vi "IR2100_get_rdg.vi"(1 "Address":T1) -> (3 "Comment":string, 5 "Reading":dbl format="%.3f")   [LabVIEW 2017]
uses:
  ADAM Client/Sub VIs/ADAM Controls/Address.ctl
  <vilib>/Instr/serial.llb/serpConfig.vi
  <vilib>/Plasmionique/MB Master/MB Master.lvlib
  <vilib>/Plasmionique/MB Master/MB_Master_Serial/MB_Master_Serial.lvclass
  Applications/National Instruments/LabVIEW 2017 64-bit/vi.lib/Plasmionique/MB Master/MB_Master/MB_Master.lvclass
panel:
  out "Results (binary)":u16[](array[numeric])
  out "error out":errorcluster
  out "Channel":u16(ring) items=["Current Value", "Mode", "Status", "Gas type", "Unit type", "Version", "Gain", "Disable LED", "Solenoid I/O", "Address", "Ratio", "Baud Rate", "Data Format", "Not Used", "Not Used", "Not Used", "Not Used", "Not Used", "Not Used", "Not Used", "Not Used", "Not Used", "Not Used", "Not Used", "Not Used", "Not Used", "Not Used", "Not Used", "Not Used", "Not Used", "Not Used", "Not Used", "# Rcv Errors", "% Activity Rate", "# Function Err", "# Start Errors", "# Register Err.", "# CRC hi Errors", "# CRC lo Errors", "# Overrun Err.", "# Noise Errors", "# Framing Err", "Not Used", "Not Used", "Not Used", "Clear Errors"]
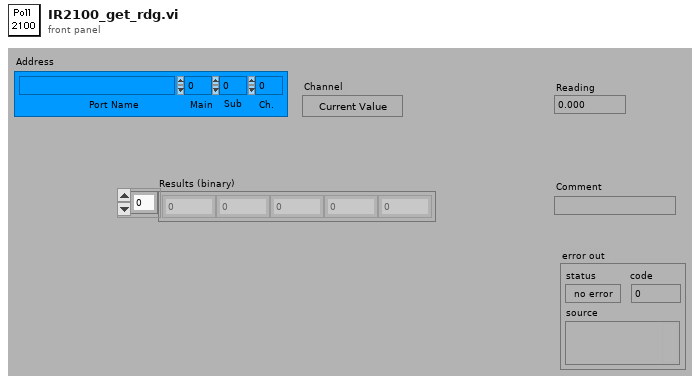
[diagram p1: front panel]
types:
  T1 = typedef "Address.ctl" = cluster{"Main":i32, "Ch.":i32, "Sub":i32, "Port Name":string}
  T2 = cluster{"baud rate (bps)":u32, "stop bits":u16, "parity":u16, "flow control":u16, "timeout":u32, "retries":i32}
  T3 = enum16{"01 Read digital output status", "02 Read digital input status", "03 Read output registers", "04 Read input registers", "05 Write single digital output", "06 Write single output register", "15 Write multiple digital outputs", "16 Write multiple output registers"}
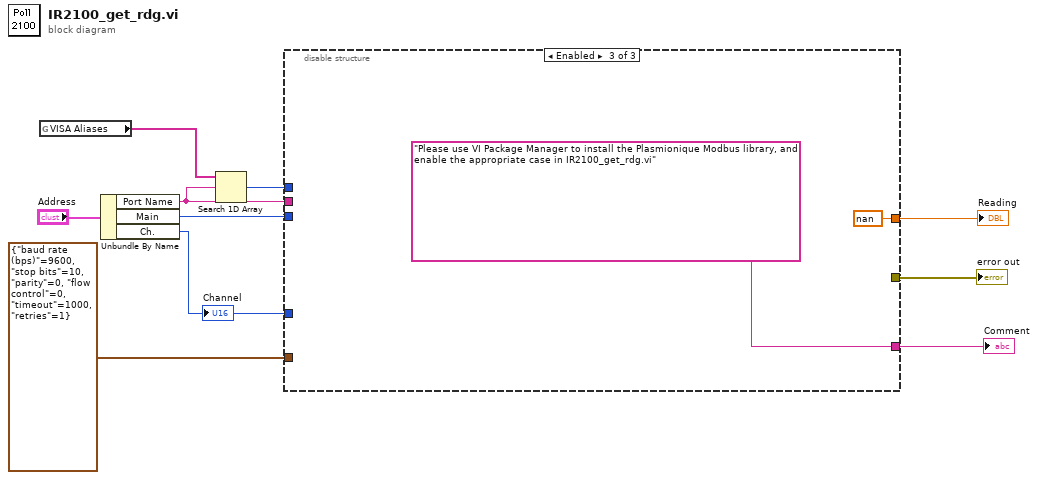
[diagram p0: block diagram]
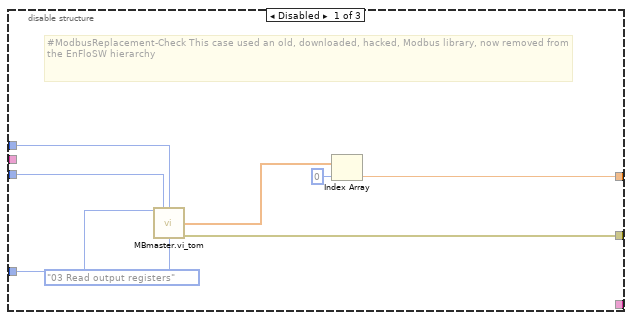
[diagram p2: hidden frame]
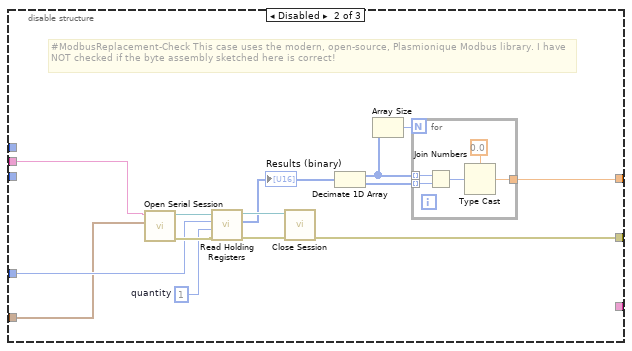
[diagram p3: hidden frame]
diagram:
  n1 = global read "serpConfig.vi" "VISA Aliases"() -> (w8:string[])
  n2 = Unbundle By Name("Address") -> ("Port Name"=w3:string, "Main"=w6:i32, "Ch."=w5:i32)
  "Channel" <- w5
  n3 = Search 1D Array(1D array=w8, element=w3) -> (index of element=w7:i32)  [unwired: 1 out]
  n4 = disable-structure shown="Enabled" {
    disable-tunnel: [w15 w20 nan ("Reading")] -> w10
    disable-tunnel: w7 -> [w14 _ _]
    disable-tunnel: w6 -> [w13 _ _]
    disable-tunnel: w5 -> [w12 w26 _]
    disable-tunnel: [w11 w30 _] -> w4
    disable-tunnel: w3 -> [_ w29 _]
    disable-tunnel: T2 {"baud rate (bps)"=9600, "stop bits"=10, "parity"=0, "flow control"=0, "timeout"=1000, "retries"=1} ("Serial Config") -> [_ w19 _]
    disable-tunnel: [_ _ "Please use VI Package Manager to install the Plasmionique Modbus library, and enable the appropriate case in IR2100_get_rdg.vi"] -> w1
    frame Disabled {
      # "#ModbusReplacement-Check This case used an old, downloaded, hacked, Modbus library, now removed from the EnFloSW hierarchy"
      n5 = call "MBmaster.vi_tom.vi"("Register address (0)"=w12, "Modbus address (1)"=w13, "port number"=w14, "ModBus Function"=T3."03 Read output registers") -> ("Process values"=w17:dbl[], "error out"=w11:errorcluster)  [unwired: 5 in, 5 out]
      n6 = Index Array(array=w17, index=0) -> (element=w15:dbl)
    }
    frame Disabled {
      w25 = u16 1  # quantity
      # "#ModbusReplacement-Check This case uses the modern, open-source, Plasmionique Modbus library. I have NOT checked if the byte assembly sketched here is correct!"
      n7 = call <vilib>:"Open Serial Session.vi"("Serial Config"=w19, "VISA Resource"=w29) -> ("Error out"=w32:errorcluster, "MB_Serial session"=w28:refnum<class "MB_Master_Serial.lvclass">)  [unwired: 8 in]
      n8 = call <vilib>:"Read Holding Registers.vi"("error in (no error)"=w32, "quantity"=w25, "starting address"=w26, "MB session in"=w28) -> ("error out"=w31:errorcluster, "Registers"=w21:u16[], "MB session out"=w27:refnum<class "MB_Master_Serial.lvclass">)  [unwired: 5 in]
      "Results (binary)" <- w21
      n9 = call-dynamic "Close Session.vi"("error in (no error)"=w31, "MB_Serial session"=w27) -> ("error out"=w30:errorcluster)  [unwired: 9 in]
      n10 = Decimate 1D Array(w21) -> (w23:u16[], w24:u16[])
      n11 = Array Size(array=w23) -> (size(s)=w22:i32)
      n12 = for {
        N: w22 -> [_]
        tunnel: w23 -> [w36] mode=indexing
        tunnel: w24 -> [w37] mode=indexing
        tunnel: [w33] -> w20
        n13 = Join Numbers(hi=w36, lo=w37) -> ((hi.lo)=w35:u32)
        n14 = Type Cast(type=sgl 0.0, x=w35) -> (*(type *) &x=w33:sgl)
      }
    }
    frame Enabled {
    }
  }
  "Reading" <- w10
  "Comment" <- w1
  "error out" <- w4
